vi "Configure Export Signal.vi"(8 "error in":errorcluster, 11 "Scope PXI CFG in":refnum<class "Scope PXI CFG.lvclass">) -> (0 "error out":errorcluster, 3 "Scope PXI CFG out":refnum<class "Scope PXI CFG.lvclass">)   [LabVIEW 2023, in "HAL.lvlib" / "Scope PXI.lvlib" / "Scope PXI CFG.lvclass"]
uses:
  Scope PXI CFG.lvclass
  Scope PXI CFG.lvclass/Scope PXI CFG.ctl
  Configuration Base/Configuration Base.lvclass
  <vilib>/Utility/error.llb/Error Cluster From Error Code.vi
  <vilib>/ErrorRing/Error Ring.xnode
  2730e925-9606-4ad7-9a46-8b9e9f9d343d.vi
  eeedd880-040e-4334-9e90-55d09acfd16d.vi
  c8bb0508-7956-418a-a24e-ae04bd9a5285.vi
  <vilib>/JDP Science/JSONtext/JSONtext.lvlib
  <instrlib>/niScope/Controls/niScope export destinations.ctl
  <instrlib>/niScope/Controls/niScope exportable signals.ctl
  D:/git/HAL/Configuration Base/Configuration Base.lvclass
  D:/git/HAL/Interfaces/IConfigure/IConfigure.lvclass
  D:/git/HAL/Scope PXI/Scope PXI CFG/Scope PXI CFG.lvclass
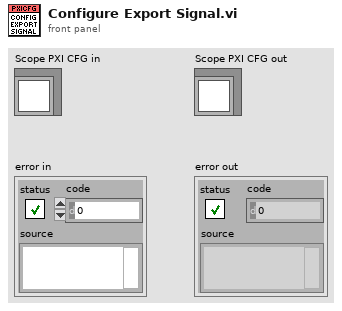
[diagram p1: front panel]
types:
  T1 = typedef "niScope export destinations.ctl" = string
  T2 = typedef "niScope exportable signals.ctl" = u16
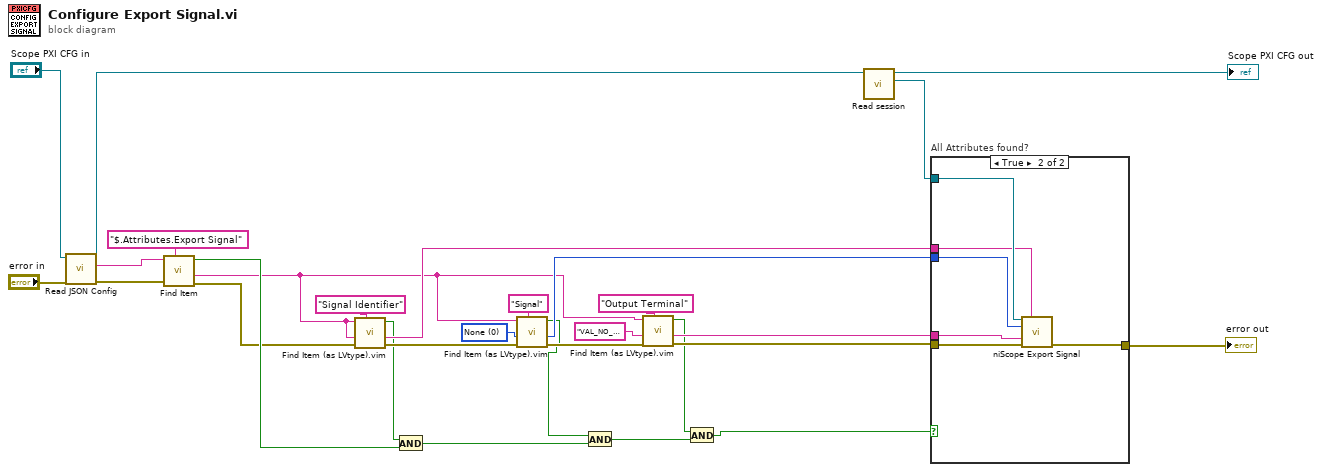
[diagram p0: block diagram]
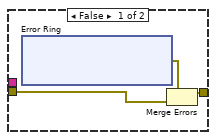
[diagram p2: hidden frame]
diagram:
  w4 = T2 0 items=["None"=0, "Start Trigger"=2, "Advance Trigger"=5, "Reference Trigger"=1, "End of Record Event"=4, "End of Acquisition Event"=3, "Ready for Start Event"=7, "Ready for Advance Event"=6, "Ready for Reference Event"=10, "Reference Clock"=100, "Sample Clock"=101, "5 Volt Power"=13] ("signal")
  n1 = call "Read JSON Config.vi"("error in"="error in", "object in"="Scope PXI CFG in") -> ("error out"=w28:errorcluster, "<JSON>Config"=w25:string, "object out"=w26:refnum<class "Scope PXI CFG.lvclass">)  [unwired: 7 in]
  n2 = call <vilib>:"Find Item.vi"("$Path or Item Name"="$.Attributes.Export Signal", "error in (no error)"=w28, "JSON"=w25) -> ("error out"=w23:errorcluster, "<JSON>"=w1:string, "Found"=w24:bool)  [unwired: 5 in, 1 out]
  n3 = call "Find Item (as LVtype).vim"("$Path or Item Name"="Signal Identifier", "error in (no error)"=w23, "Data Type and Default Value"=w1, "JSON"=w1) -> ("error out"=w20:errorcluster, "Data"=w19:string, "Found"=w13:bool)  [unwired: 4 in, 1 out]
  n4 = And(x=w13, y=w24) -> (x .and. y?=w11:bool)
  n5 = call "Find Item (as LVtype).vim"("$Path or Item Name"="Signal", "error in (no error)"=w20, "Data Type and Default Value"=w4, "JSON"=w1) -> ("error out"=w16:errorcluster, "Data"=w18:T2, "Found"=w12:bool)  [unwired: 4 in, 1 out]
  n6 = And(x=w12, y=w11) -> (x .and. y?=w9:bool)
  n7 = call "Find Item (as LVtype).vim"("$Path or Item Name"="Output Terminal", "error in (no error)"=w16, "Data Type and Default Value"=T1 "VAL_NO_SOURCE" ("output terminal"), "JSON"=w1) -> ("error out"=w15:errorcluster, "Data"=w14:T1, "Found"=w10:bool)  [unwired: 4 in, 1 out]
  n8 = And(x=w10, y=w9) -> (x .and. y?=w2:bool)
  n9 = call "Read session.vi"("Scope PXI CFG in"=w26) -> ("session"=w27:refnum<k15>, "Scope PXI CFG out"=→"Scope PXI CFG out":refnum<class "Scope PXI CFG.lvclass">)  [unwired: 8 in, 1 out]
  n10 = case "All Attributes found?" shown="True" w2 {
    tunnel: w15 -> [w30 w42]
    tunnel: w19 -> [_ w40]
    tunnel: w18 -> [_ w39]
    tunnel: [w31 w41] -> w6
    tunnel: w14 -> [_ w38]
    tunnel: w27 -> [_ w43]
    frame False {
      n11 = xnode "Error Ring"() -> ("error out"=w32:errorcluster)
      n12 = Merge Errors(w32, w30) -> (w31:errorcluster)
    }
    frame True {
      n13 = call <instrlib>:"niScope Export Signal.vi"("instrument handle"=w43, "signal identifier"=w40, "signal"=w39, "output terminal"=w38, "error in"=w42) -> ("error out"=w41:errorcluster)  [unwired: 9 in, 1 out]
    }
  }
  "error out" <- w6
